vi "Excel Integration.vi"() -> ()   [LabVIEW 2015]
uses:
  <vilib>/Utility/file.llb/Write Delimited Spreadsheet (string).vi
  <vilib>/Utility/file.llb/Write Delimited Spreadsheet (DBL).vi
panel:
  out "FAILED":bool
  out "Completed":bool
  out "?":string
  out "Heading":string
  in  "Text file path":path
  in  "S.N.":i32
  out "S.N                       First                     Last":dbl[](array[numeric])
  in  "Stop":bool
  out "Heading":string[](array[string])
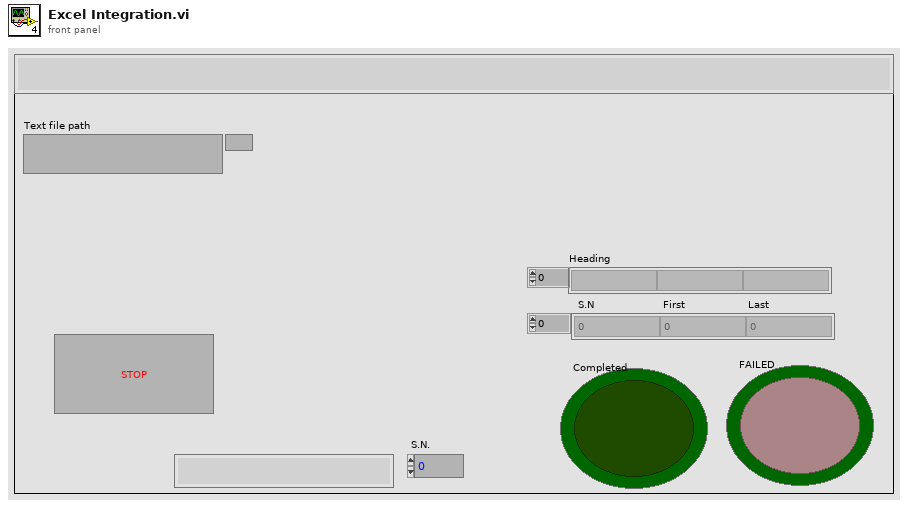
[diagram p1: front panel]
types:
  T1 = enum16{"open", "replace", "create", "open or create", "replace or create", "replace or create with confirmation"}
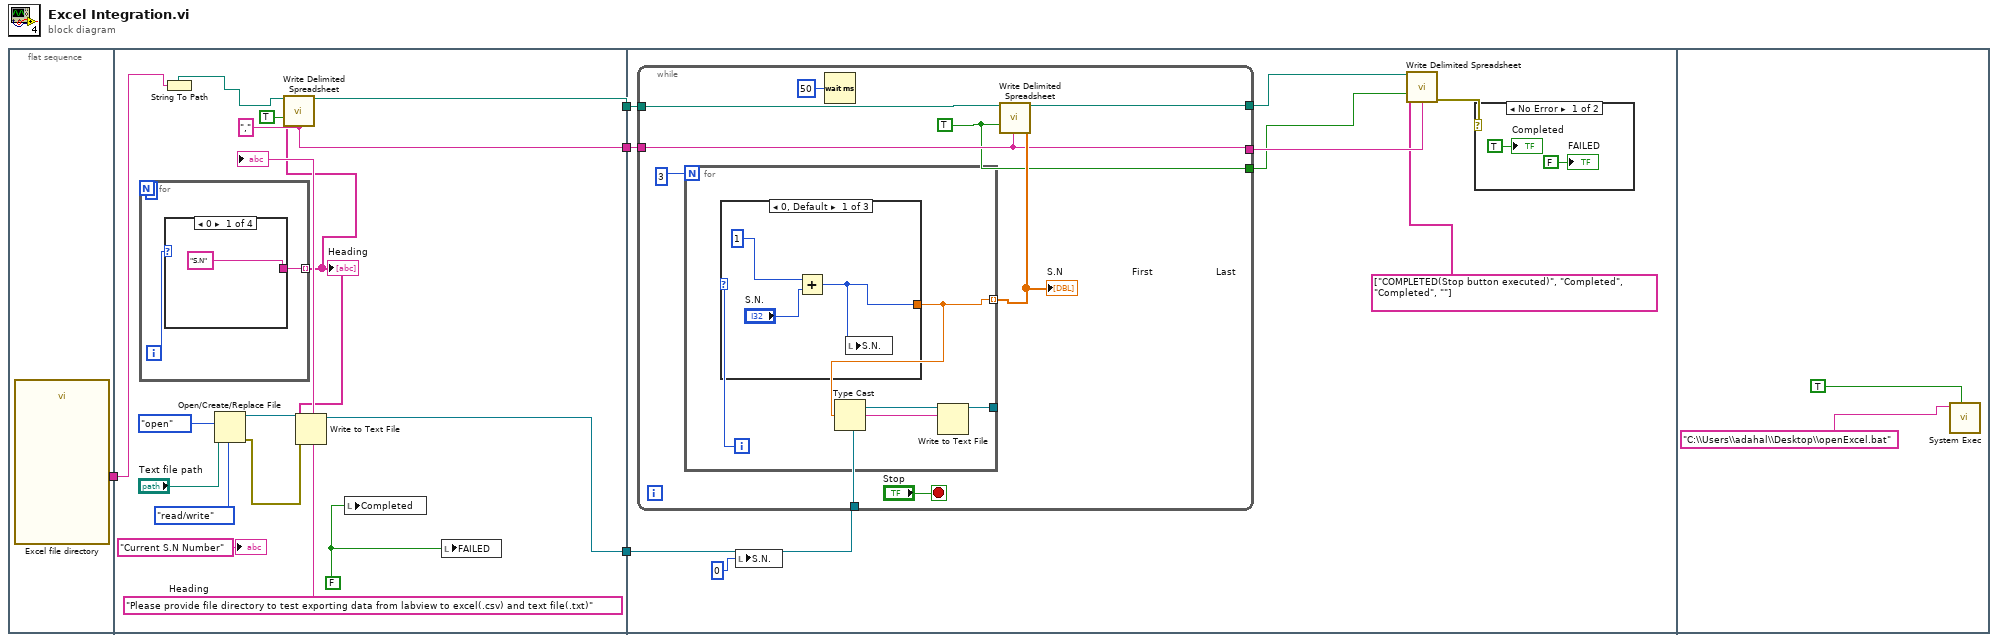
[diagram p0: block diagram]
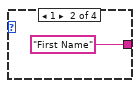
[diagram p2: hidden frame]
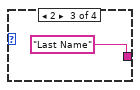
[diagram p3: hidden frame]
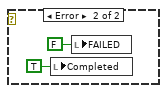
[diagram p5: hidden frame]
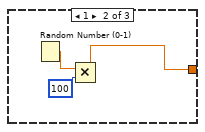
[diagram p6: hidden frame]
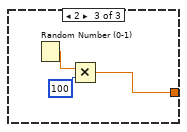
[diagram p7: hidden frame]
diagram:
  n1 = flat-sequence {
    tunnel: [w5] -> w1
    tunnel: [w19] -> w4
    tunnel: [w20] -> w3
    tunnel: [w8] -> w2
    tunnel: w1 -> [w7]
    tunnel: w4 -> [w35]
    tunnel: w3 -> [w34]
    tunnel: w2 -> [w27]
    frame #0 {
      n2 = call "Excel file directory"() -> ("Path:"=w5:string)  [unwired: 17 in, 2 out]
    }
    frame #1 {
      w10 = FALSE ("Completed")
      w20 = "," ("delimiter (\\t)")
      n3 = for {
        N: 3 -> [_]
        tunnel: [w22] -> w11 mode=indexing
        i -> [w23]
        n4 = case shown="0" w23 {
          tunnel: ["S.N" "First Name" "Last Name" _] -> w22
          frame 0 {
          }
          frame 1 {
          }
          frame 2 {
          }
          frame 3, Default {
          }
        }
      }
      "Heading" <- w11
      n5 = String To Path(string=w7) -> (path=w6:path)
      n6 = Open/Create/Replace File(file path (use dialog)="Text file path", operation (0:open)=T1."open", access (0:read/write)=enum16{"read/write", "read-only", "write-only"}."read/write") -> (refnum out=w15:refnum<file>, error out=w16:errorcluster)  [unwired: 3 in, 1 out]
      n7 = call-poly <vilib>:"Write Delimited Spreadsheet.vi"("file path (dialog if empty)"=w6, "1D data"=w11, "append to file? (F)"=TRUE, "delimiter (\\t)"=w20) -> ("new file path (Not A Path if cancelled)"=w19:path)  [unwired: 10 in, 1 out]
      n8 = Write to Text File(file (use dialog)=w15, text=w11, error in=w16) -> (refnum out=w8:refnum<file>)  [unwired: 1 in, 2 out]
      n9 = local write "Completed"(w10) -> ()
      n10 = local write "FAILED"(w10) -> ()
      "Heading" <- "Please provide file directory to test exporting data from labview to excel(.csv) and text file(.txt)" ("Heading")
      "?" <- "Current S.N Number"
    }
    frame #2 {
      n11 = while {
        tunnel: w35 -> [w42]
        tunnel: w34 -> [w44]
        tunnel: [w44] -> w32
        tunnel: [w43] -> w29
        tunnel: [w41] -> w31
        tunnel: w27 -> [w40]
        stop <- "Stop" stop-if-true
        w43 = TRUE ("append to file? (F)")
        n12 = for {
          N: 3 -> [_]
          tunnel: [w50] -> w45 mode=indexing
          tunnel: w40 -> [w51]
          i -> [w52]
          n13 = case shown="0, Default" w52 {
            tunnel: [w53 w56 w59] -> w50
            frame 0, Default {
              n14 = Add(x=1, y="S.N.") -> (x+y=w53:i32)
              n15 = local write "S.N."(w53) -> ()
            }
            frame 1 {
              n16 = Random Number (0-1)() -> (number: 0 to 1=w57:dbl)
              n17 = Multiply(x=w57, y=100) -> (x*y=w56:dbl)
            }
            frame 2 {
              n18 = Random Number (0-1)() -> (number: 0 to 1=w61:dbl)
              n19 = Multiply(x=w61, y=100) -> (x*y=w59:dbl)
            }
          }
          n20 = Type Cast(x=w50) -> (*(type *) &x=w49:string)  [unwired: 1 in]
          n21 = Write to Text File(file (use dialog)=w51, text=w49) -> ()  [unwired: 2 in, 3 out]
        }
        "S.N                       First                     Last" <- w45
        n22 = Wait (ms)(milliseconds to wait=u32 50) -> ()  [unwired: 1 out]
        n23 = call-poly <vilib>:"Write Delimited Spreadsheet.vi"("file path (dialog if empty)"=w42, "1D data"=w45, "append to file? (F)"=w43, "delimiter (\\t)"=w44) -> ("new file path (Not A Path if cancelled)"=w41:path)  [unwired: 10 in, 1 out]
      }
      n24 = local write "S.N."(0 ("Numeric")) -> ()
      n25 = call-poly <vilib>:"Write Delimited Spreadsheet.vi"("file path (dialog if empty)"=w31, "1D data"=string[] ["COMPLETED(Stop button executed)", "Completed", "Completed", ""], "append to file? (F)"=w29, "delimiter (\\t)"=w32) -> ("error out"=w28:errorcluster)  [unwired: 10 in, 1 out]
      n26 = case shown="No Error" w28 {
        frame No Error {
          "Completed" <- TRUE ("Boolean")
          "FAILED" <- FALSE ("Boolean 2")
        }
        frame Error {
          n27 = local write "Completed"(TRUE ("Completed")) -> ()
          n28 = local write "FAILED"(FALSE ("FAILED")) -> ()
        }
      }
    }
    frame #3 {
      n29 = call <vilib>:"System Exec.vi"("wait until completion? (T)"=TRUE, "command line"="C:\\Users\\adahal\\Desktop\\openExcel.bat" ("standard input")) -> ()  [unwired: 6 in, 4 out]
    }
  }
